vi "GaussanalysisCK.vi"(8 "Image":T3, 9 "Y parameter bounds":T2={"amp min"=-inf, "amp max"=inf, "center min"=-inf, "center max"=inf, "deviation min"=-inf, "deviation max"=inf, "offset min"=0.0, "offset max"=0.0}, 10 "X parameter bounds":T2={"amp min"=-inf, "amp max"=inf, "center min"=-inf, "center max"=inf, "deviation min"=-inf, "deviation max"=inf, "offset min"=0.0, "offset max"=0.0}) -> (1 "Fit successful":bool, 2 "Cluster":T1, 3 "XY Graph":cluster{i32[], "Best Gaussian Fit":dbl[]}[](graph))   [LabVIEW 2009]
uses:
  <vilib>/vision/Image Controls.llb/IMAQ Image.ctl
  <vilib>/vision/NI_Vision_Development_Module.lvlib
  <vilib>/Analysis/NI_AALPro.lvlib
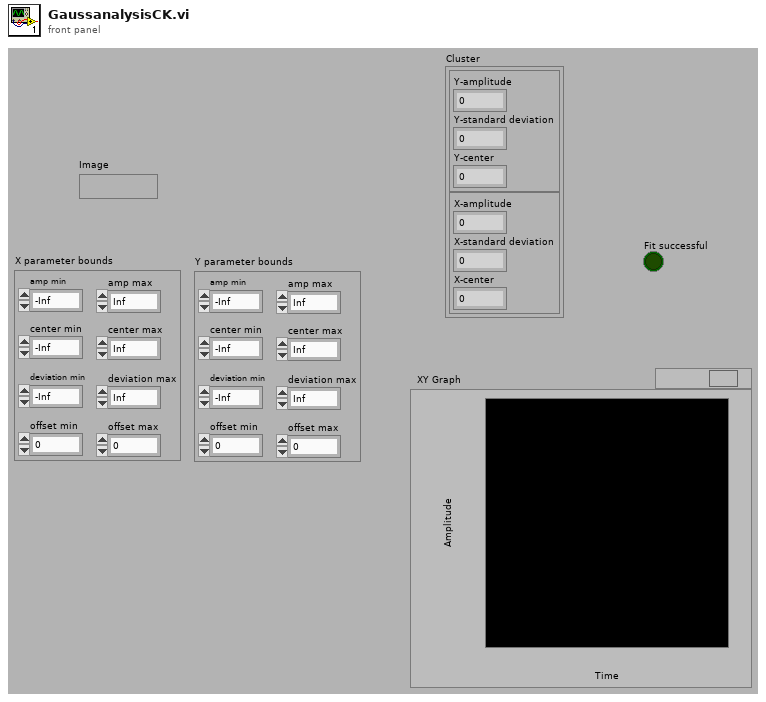
[diagram p1: front panel]
types:
  T1 = cluster{cluster{"Y-amplitude":dbl, "Y-standard deviation":dbl, "Y-center":dbl}, cluster{"X-amplitude":dbl, "X-standard deviation":dbl, "X-center":dbl}}
  T2 = cluster{"amp min":dbl, "amp max":dbl, "center min":dbl, "center max":dbl, "deviation min":dbl, "deviation max":dbl, "offset min":dbl, "offset max":dbl}
  T3 = typedef "IMAQ Image.ctl" = refnum<image>
  T4 = cluster{"amplitude":dbl, "standard deviation":dbl, "center":dbl}
  T5 = cluster{cluster{"amplitude":dbl, "standard deviation":dbl, "center":dbl}, cluster{"amplitude":dbl, "standard deviation":dbl, "center":dbl}}
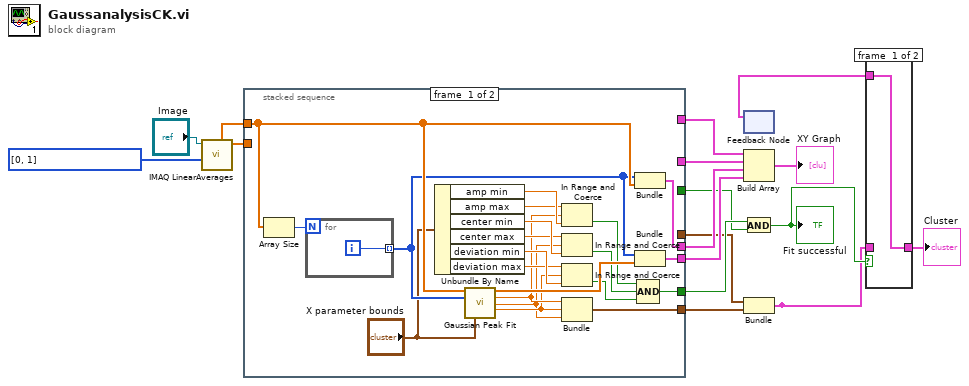
[diagram p0: block diagram]
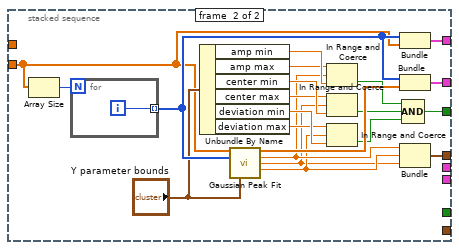
[diagram p3: hidden frame]
diagram:
  w12 = i32[] [0, 1] items=["X Axis Averages", "Y Axis Averages", "X + Y Axis Averages", "X - Y Axis Averages"] ("Averages")
  n1 = call "IMAQ LinearAverages"("Averages"=w12, "Image Src"="Image") -> ("Y Axis Averages"=w10:sgl[], "X Axis Averages"=w9:sgl[])  [unwired: 5 in, 3 out]
  n2 = stacked-sequence {
    tunnel: [_ w41] -> w13
    tunnel: [_ w40] -> w14
    tunnel: [w38 _] -> w15
    tunnel: [w37 _] -> w16
    tunnel: w10 -> [_ w44]
    tunnel: w9 -> [w35 _]
    tunnel: [w19 _] -> w5
    tunnel: [w18 _] -> w8
    tunnel: [_ w43] -> w7
    tunnel: [_ w42] -> w6
    frame #0 {
      n3 = Array Size(array=w35) -> (size(s)=w36:i32)
      n4 = for {
        N: w36 -> [_]
        tunnel: [w39] -> w34 mode=indexing
        i -> [w39]
      }
      n5 = Unbundle By Name("X parameter bounds") -> ("amp min"=w31:dbl, "amp max"=w30:dbl, "center min"=w29:dbl, "center max"=w28:dbl, "deviation min"=w27:dbl, "deviation max"=w26:dbl)
      n6 = call <vilib>:"Gaussian Peak Fit.vi"("Y"=w35, "X"=w34, "parameter bounds"="X parameter bounds") -> ("Best Gaussian Fit"=w33:dbl[], "amplitude"=w22:dbl, "center"=w20:dbl, "standard deviation"=w21:dbl)  [unwired: 6 in, 3 out]
      n7 = In Range and Coerce(upper limit=w30, x=w22, lower limit=w31) -> (In Range?=w25:bool)  [unwired: 1 out]
      n8 = In Range and Coerce(upper limit=w28, x=w20, lower limit=w29) -> (In Range?=w24:bool)  [unwired: 1 out]
      n9 = In Range and Coerce(upper limit=w26, x=w21, lower limit=w27) -> (In Range?=w23:bool)  [unwired: 1 out]
      n10 = Bundle("amplitude"=w22, "standard deviation"=w21, "center"=w20) -> (w19:T4)  [unwired: 1 in]
      n11 = Bundle(w34, "X Axis Averages"=w35) -> (w38:cluster{i32[], "X Axis Averages":sgl[]})  [unwired: 1 out]
      n12 = Bundle(w34, "Best Gaussian Fit"=w33) -> (w37:cluster{i32[], "Best Gaussian Fit":dbl[]})  [unwired: 1 out]
      n13 = Compound Arithmetic op=AND(w25, w24, w23) -> (w18:bool)
    }
    frame #1 {
      n14 = Array Size(array=w44) -> (size(s)=w60:i32)
      n15 = for {
        N: w60 -> [_]
        tunnel: [w61] -> w59 mode=indexing
        i -> [w61]
      }
      n16 = Unbundle By Name("Y parameter bounds") -> ("amp min"=w56:dbl, "amp max"=w55:dbl, "center min"=w54:dbl, "center max"=w53:dbl, "deviation min"=w52:dbl, "deviation max"=w51:dbl)
      n17 = call <vilib>:"Gaussian Peak Fit.vi"("Y"=w44, "X"=w59, "parameter bounds"="Y parameter bounds") -> ("Best Gaussian Fit"=w58:dbl[], "amplitude"=w47:dbl, "center"=w45:dbl, "standard deviation"=w46:dbl)  [unwired: 6 in, 3 out]
      n18 = In Range and Coerce(upper limit=w55, x=w47, lower limit=w56) -> (In Range?=w50:bool)  [unwired: 1 out]
      n19 = In Range and Coerce(upper limit=w53, x=w45, lower limit=w54) -> (In Range?=w49:bool)  [unwired: 1 out]
      n20 = In Range and Coerce(upper limit=w51, x=w46, lower limit=w52) -> (In Range?=w48:bool)  [unwired: 1 out]
      n21 = Bundle(w59, "Y Axis Averages"=w44) -> (w41:cluster{i32[], "Y Axis Averages":sgl[]})  [unwired: 1 out]
      n22 = Bundle(w59, "Best Gaussian Fit"=w58) -> (w40:cluster{i32[], "Best Gaussian Fit":dbl[]})  [unwired: 1 out]
      n23 = Bundle("amplitude"=w47, "standard deviation"=w46, "center"=w45) -> (w42:T4)  [unwired: 1 in]
      n24 = Compound Arithmetic op=AND(w50, w49, w48) -> (w43:bool)
    }
  }
  n25 = feedback #1() -> (w1:T5)  [unwired: 1 in]
  n26 = Build Array(w13, w14, w15, w16) -> (→"XY Graph":cluster{i32[], "Best Gaussian Fit":dbl[]}[])
  n27 = And(x=w8, y=w7) -> (x .and. y?=w3:bool)
  "Fit successful" <- w3
  n28 = Bundle(w6, w5) -> (w2:T5)  [unwired: 1 in]
  n29 = case shown="False" w3 {
    tunnel: [w62 w63] -> w4
    tunnel: w2 -> [_ w63]
    tunnel: w1 -> [w62 _]
    frame #0 {
    }
    frame #1 {
    }
  }
  "Cluster" <- w4
